vi "User Access Level FGV Unit Test_EX.vi"() -> ()   [LabVIEW 2021]
uses:
  UserLevel.ctl
panel:
  in  "Access Secure Area":bool
  out "Error Out":errorcluster
  in  "Error In":errorcluster
  in  "Current User":string
  in  "Set User Access Level":bool
  in  "stop":bool
  # "1.  Set access level for current user."
  # "2.  Test access level by verifying the appropriate dialog message."
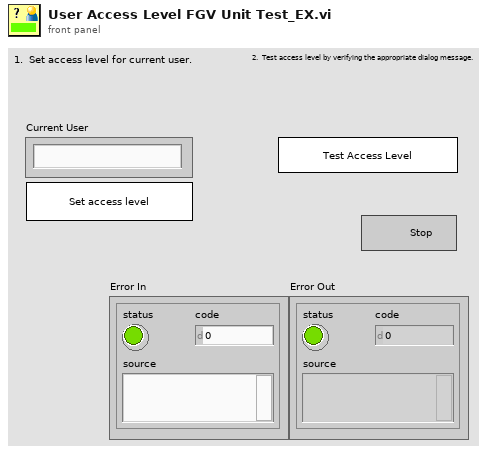
[diagram p1: front panel]
types:
  T1 = typedef "UserLevel.ctl" = enum16{"Read User Access Level File", "Set Current User", "Get User Access Level"}
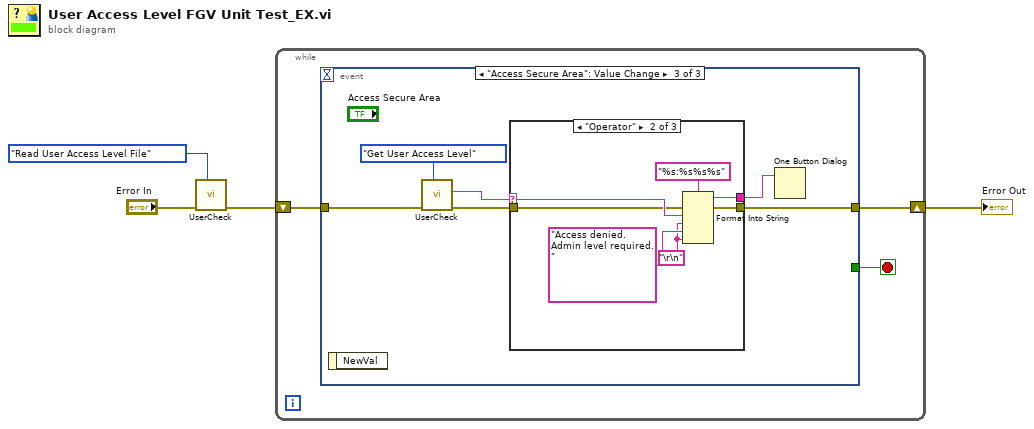
[diagram p0: block diagram]
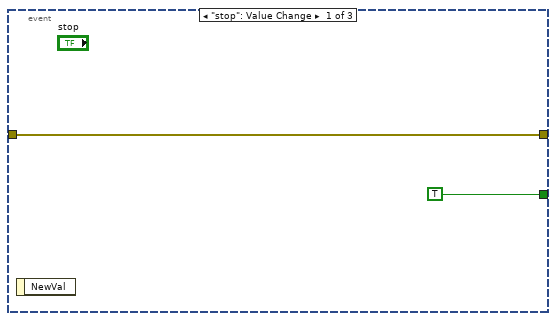
[diagram p2: hidden frame]
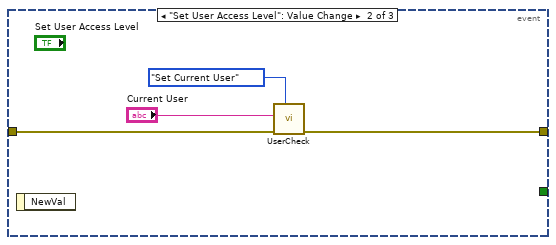
[diagram p3: hidden frame]
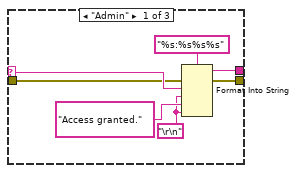
[diagram p4: hidden frame]
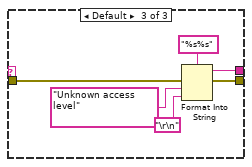
[diagram p5: hidden frame]
diagram:
  n1 = call "UserCheck.vi"("Enum"=UserLevel."Read User Access Level File", "error in (no error)"="Error In") -> ("error out"=w4:errorcluster)  [unwired: 8 in, 1 out]
  n2 = while {
    shift-right: [w5] -> w2
    shift-left: w4 -> [w6]
    stop <- w7 stop-if-true
    n3 = event shown="[2] \"Access Secure Area\": Value Change" {
      selector: _ -> [_ _ _]
      dyn-events: _ -> [_ _ _]
      timeout: _ -> [_ _ _]
      tunnel: [TRUE ("stop") _ _] -> w7
      tunnel: w6 -> [w8 w13 w19]
      tunnel: [w8 w11 w18] -> w5
      event "stop": Value Change {
        n4 = event-data() -> ()  [unwired: 1 in, 1 out]
      }
      event "Set User Access Level": Value Change {
        n5 = event-data() -> ()  [unwired: 1 in, 1 out]
        n6 = call "UserCheck.vi"("Enum"=UserLevel."Set Current User", "error in (no error)"=w13, "User Name"="Current User") -> ("error out"=w11:errorcluster)  [unwired: 7 in, 1 out]
      }
      event "Access Secure Area": Value Change {
        n7 = event-data() -> ()  [unwired: 1 in, 1 out]
        n8 = call "UserCheck.vi"("Enum"=UserLevel."Get User Access Level", "error in (no error)"=w19) -> ("error out"=w17:errorcluster, "User Level"=w16:string)  [unwired: 8 in]
        n9 = case shown="\"Operator\"" w16 {
          selector: w16 -> [w26 w33 _]
          tunnel: [w24 w31 w38] -> w18
          tunnel: w17 -> [w25 w32 w39]
          tunnel: [w20 w27 w36] -> w15
          frame "Admin" {
            w22 = "\r\n"
            n10 = Format Into String(format string="%s:%s%s%s", error in=w25, w26, w22, "Access granted." ("message"), w22) -> (resulting string=w20:string, error out=w24:errorcluster)  [unwired: 1 in]
          }
          frame "Operator" {
            w29 = "\r\n"
            n11 = Format Into String(format string="%s:%s%s%s", error in=w32, w33, w29, "Access denied.  Admin level required." ("message"), w29) -> (resulting string=w27:string, error out=w31:errorcluster)  [unwired: 1 in]
          }
          frame Default {
            n12 = Format Into String(format string="%s%s", error in=w39, "Unknown access level" ("message"), "\r\n") -> (resulting string=w36:string, error out=w38:errorcluster)  [unwired: 1 in]
          }
        }
        n13 = One Button Dialog(message=w15) -> ()  [unwired: 1 in, 1 out]
      }
    }
  }
  "Error Out" <- w2
